vi "SHA1.vi"(1 "String":string) -> (0 "SHA1":string)   [LabVIEW 2023]
panel:
  # "\"\" => da39a3ee5e6b4b0d3255bfef95601890afd80709"
  # "The quick brown fox jumps over the lazy dog =>\n2fd4e1c67a2d28fced849ee1bb76e7391b93eb12"
  # "The quick brown fox jumps over the lazy cog =>\nde9f2c7fd25e1b3afad3e85a0bd17d9b100db4b3"
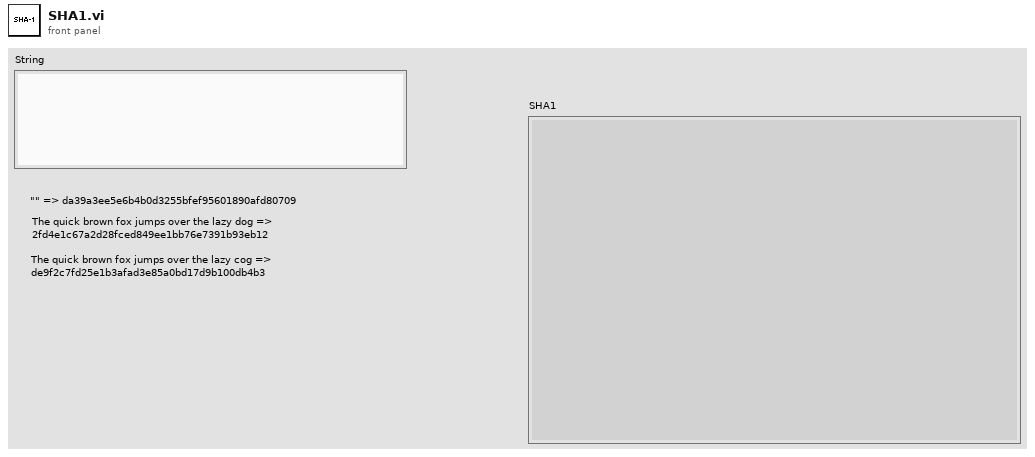
[diagram p1: front panel]
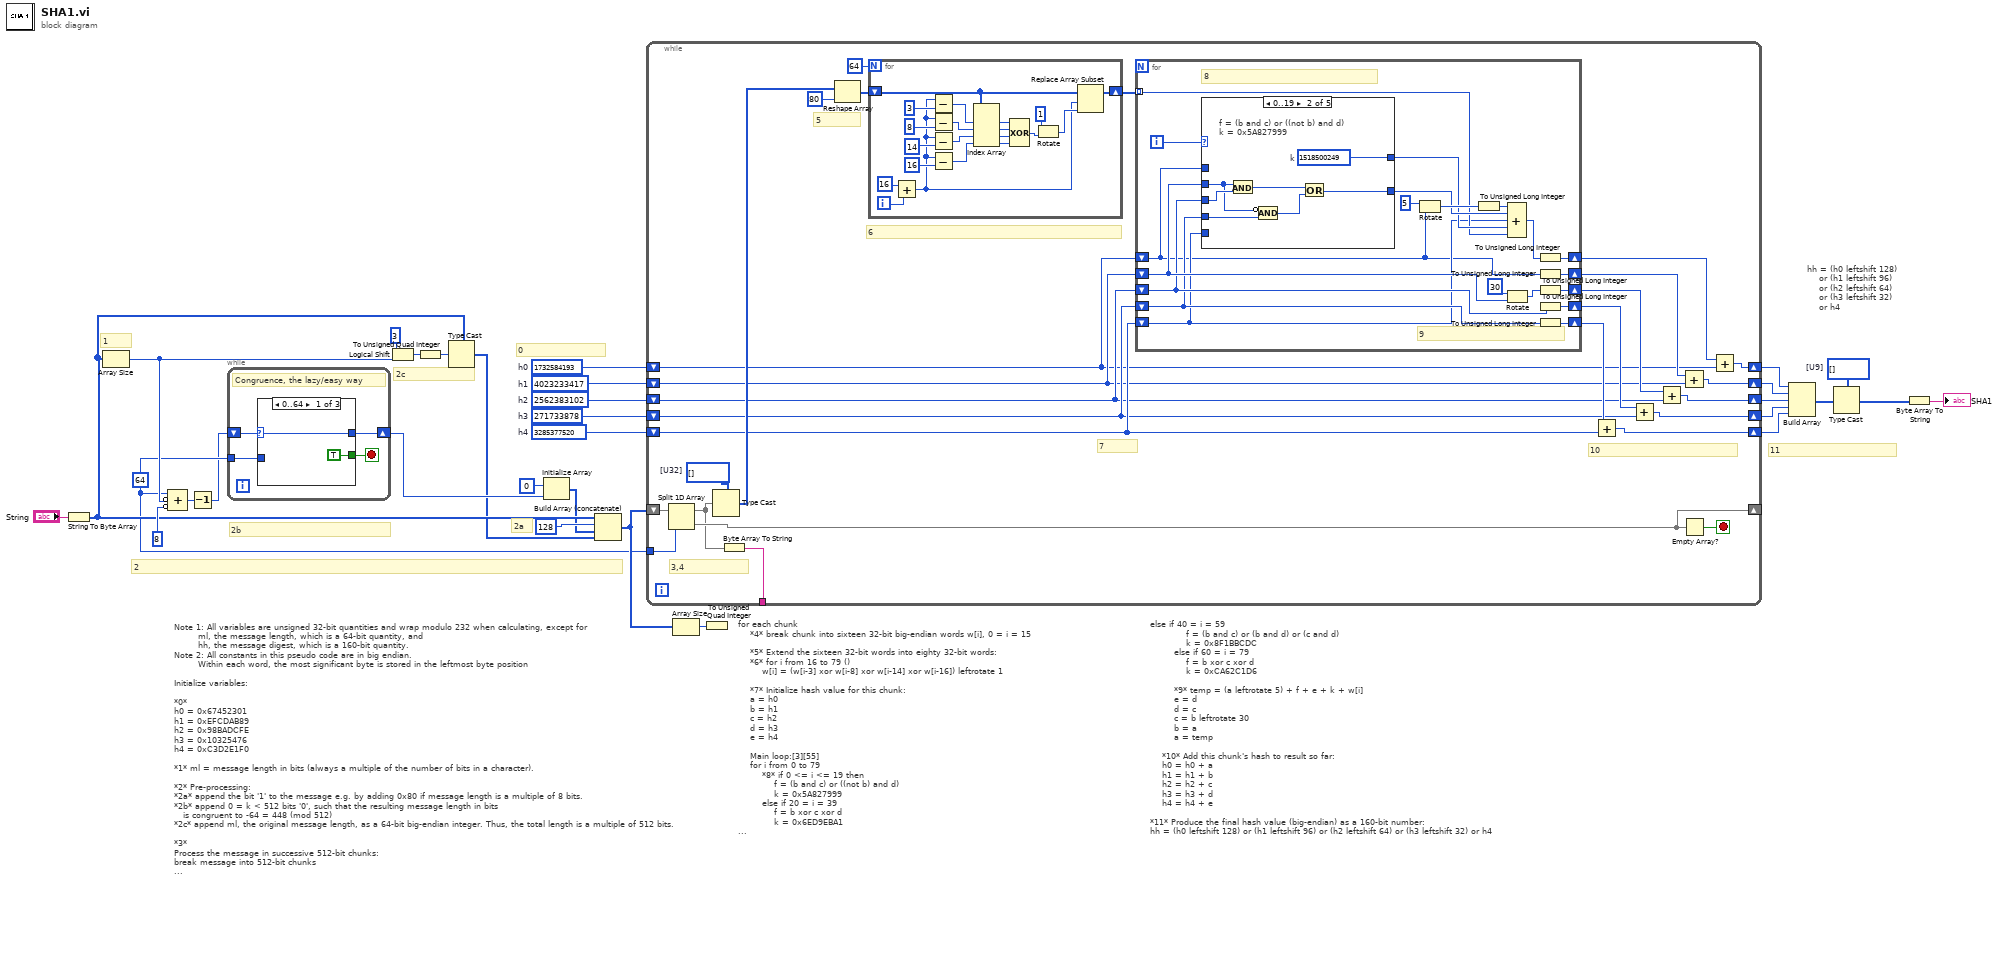
[diagram p0: block diagram]
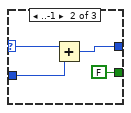
[diagram p2: hidden frame]
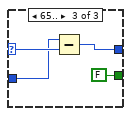
[diagram p3: hidden frame]
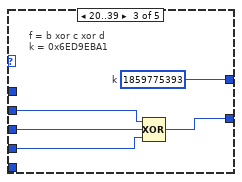
[diagram p5: hidden frame]
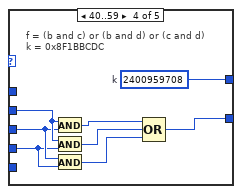
[diagram p6: hidden frame]
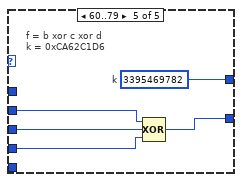
[diagram p7: hidden frame]
diagram:
  w14 = u8[] []  # [U9]
  w4 = 64 ("y")
  w22 = u32 3285377520  # h4
  w23 = u32 271733878  # h3
  w24 = u32 2562383102  # h2
  w25 = u32 4023233417  # h1
  w26 = u32 1732584193  # h0
  # "2c"
  # "2b"
  # "2a"
  # "11"
  # "hh = (h0 leftshift 128) \n    or (h1 leftshift 96) \n    or (h2 leftshift 64) \n    or (h3 leftshift 32) \n    or h4"
  # "2"
  # "1"
  # "0"
  # "else if 40 = i = 59\n            f = (b and c) or (b and d) or (c and d) \n            k = 0x8F1BBCDC\n        else if 60 = i = 79\n            f = b xor c xor d\n            k = 0xCA62C1D6\n\n        *9* temp = (a leftrotate 5) + f + e + k + w[i]\n        e = d\n        d = c\n        c = b leftrotate 30\n        b = a\n        a = temp\n\n    *10* Add this chunk's hash to result so far:\n    h0 = h0 + a\n    h1 = h1 + b \n    h2 = h2 + c\n    h3 = h3 + d\n    h4 = h4 + e\n\n*11* Produce the final hash value (big-endian) as a 160-bit number:\nhh = (h0 leftshift 128) or (h1 leftshift 96) or (h2 leftshift 64) or (h3 leftshift 32) or h4"
  # "for each chunk\n    *4* break chunk into sixteen 32-bit big-endian words w[i], 0 = i = 15\n\n    *5* Extend the sixteen 32-bit words into eighty 32-bit words:\n    *6* for i from 16 to 79 ()\n        w[i] = (w[i-3] xor w[i-8] xor w[i-14] xor w[i-16]) leftrotate 1\n\n    *7* Initialize hash value for this chunk:\n    a = h0\n    b = h1\n    c = h2\n    d = h3\n    e = h4\n\n    Main loop:[3][55]\n    for i from 0 to 79\n        *8* if 0 <= i <= 19 then\n            f = (b and c) or ((not b) and d)\n            k = 0x5A827999\n        else if 20 = i = 39\n            f = b xor c xor d\n            k = 0x6ED9EBA1\n..."
  # "Note 1: All variables are unsigned 32-bit quantities and wrap modulo 232 when calculating, except for\n        ml, the message length, which is a 64-bit quantity, and\n        hh, the message digest, which is a 160-bit quantity.\nNote 2: All constants in this pseudo code are in big endian.\n        Within each word, the most significant byte is stored in the leftmost byte position\n\nInitialize variables:\n\n*0*\nh0 = 0x67452301\nh1 = 0xEFCDAB89\nh2 = 0x98BADCFE\nh3 = 0x10325476\nh4 = 0xC3D2E1F0\n\n*1* ml = message length in bits (always a multiple of the number of bits in a character).\n\n*2* Pre-processing:\n*2a* append the bit '1' to the message e.g. by adding 0x80 if message length is a multiple of 8 bits.\n*2b* append 0 = k < 512 bits '0', such that the resulting message length in bits\n   is congruent to -64 = 448 (mod 512)\n*2c* append ml, the original message length, as a 64-bit big-endian integer. Thus, the total length is a multiple of 512 bits.\n\n*3*\nProcess the message in successive 512-bit chunks:\nbreak message into 512-bit chunks\n..."
  n1 = String To Byte Array(string="String") -> (unsigned byte array=w12:u8[])
  n2 = Array Size(array=w12) -> (size(s)=w5:i32)
  n3 = Compound Arithmetic op=ADD(w4, invert w5, invert 8 ("y")) -> (w30:i32)
  n4 = Decrement(x=w30) -> (x-1=w3:i32)
  n5 = while {
    shift-right: [w33] -> w2
    shift-left: w3 -> [w35]
    tunnel: w4 -> [w34]
    stop <- w32 stop-if-true
    # "Congruence, the lazy/easy way"
    n6 = case shown="0..64" w35 {
      selector: w35 -> [w37 w41 w45]
      tunnel: w34 -> [_ w40 w44]
      tunnel: [w37 w39 w43] -> w33
      tunnel: [TRUE FALSE FALSE] -> w32
      frame 0..64 {
      }
      frame ..-1 {
        n7 = Add(x=w41, y=w40) -> (x+y=w39:i32)
      }
      frame 65.. {
        n8 = Subtract(x=w44, y=w45) -> (x-y=w43:i32)
      }
    }
  }
  n9 = Logical Shift(y=i16 3, x=w5) -> (x << y=w7:i32)
  n10 = To Unsigned Quad Integer(1:w7) -> (0:w28:u64)
  n11 = Type Cast(type=w12, x=w28) -> (*(type *) &x=w1:u8[])
  n12 = Initialize Array(u8 0 ("h0"), w2) -> (w10:u8[])
  n13 = Build Array (concatenate)(w12, u8 128 ("h0"), w10, w1) -> (w9:u8[])
  n14 = while {
    shift-right: [w69] -> _
    shift-left: w9 -> [w72]
    tunnel: w4 -> [w46]
    shift-right: [w68] -> w19
    shift-left: w26 -> [w49]
    shift-right: [w67] -> w18
    shift-left: w25 -> [w50]
    shift-right: [w66] -> w20
    shift-left: w24 -> [w51]
    shift-right: [w65] -> w17
    shift-left: w23 -> [w52]
    shift-right: [w64] -> w21
    shift-left: w22 -> [w53]
    tunnel: [w47] -> _
    stop <- w71 stop-if-true
    w70 = u32[] []  # [U32]
    # "10"
    # "7"
    # "5"
    # "6"
    # "3,4"
    n15 = Split 1D Array(array=w72, index=w46) -> (first subarray=w48:u8[], second subarray=w69:u8[])
    n16 = Type Cast(type=w70, x=w48) -> (*(type *) &x=w58:u32[])
    n17 = Byte Array To String(unsigned byte array=w48) -> (string=w47:string)
    n18 = Reshape Array(w58, 80 ("h0")) -> (w61:u32[])
    n19 = for {
      N: 64 ("h0") -> [_]
      shift-right: [w136] -> w60
      shift-left: w61 -> [w135]
      i -> [w137]
      n20 = Add(x=16 ("h0"), y=w137) -> (x+y=w118:i32)
      n21 = Subtract(x=w118, y=3 ("h0")) -> (x-y=w122:i32)
      n22 = Subtract(x=w118, y=8 ("h0")) -> (x-y=w121:i32)
      n23 = Subtract(x=w118, y=14 ("h0")) -> (x-y=w120:i32)
      n24 = Subtract(x=w118, y=16 ("h0")) -> (x-y=w119:i32)
      n25 = Index Array(array=w135, index #1=w122, index #2=w121, index #3=w120, index #4=w119) -> (element #1=w128:u32, element #2=w129:u32, element #3=w127:u32, element #4=w126:u32)
      n26 = Compound Arithmetic op=XOR(w128, w129, w127, w126) -> (w125:u32)
      n27 = Rotate(1:w125, 2:1 ("h0")) -> (0:w123:u32)
      n28 = Replace Array Subset(array=w135, new element=w123, index=w118) -> (w136:u32[])
    }
    n29 = for {
      tunnel: w60 -> [w88] mode=indexing
      shift-right: [w86] -> w54
      shift-left: w49 -> [w73]
      shift-right: [w82] -> w57
      shift-left: w53 -> [w76]
      shift-right: [w83] -> w59
      shift-left: w52 -> [w77]
      shift-right: [w84] -> w56
      shift-left: w51 -> [w78]
      shift-right: [w85] -> w55
      shift-left: w50 -> [w79]
      i -> [w92]
      # "9"
      # "8"
      n30 = case shown="0..19" w92 {
        tunnel: w73 -> [_ _ _ _ _]
        tunnel: w79 -> [_ w93 w103 w110 w115]
        tunnel: w78 -> [_ w97 w102 w109 w114]
        tunnel: w77 -> [_ w96 w101 w108 w113]
        tunnel: w76 -> [_ _ _ _ _]
        tunnel: [_ w95 w100 w111 w116] -> w90
        tunnel: [_ w94 w104 w112 w117] -> w89
        frame Default {
        }
        frame 0..19 {
          w94 = u32 1518500249  # k
          # "f = (b and c) or ((not b) and d)\nk = 0x5A827999"
          n31 = And(x=w93, y=w97) -> (x .and. y?=w98:u32)
          n32 = Compound Arithmetic op=AND(invert w93, w96) -> (w99:u32)
          n33 = Or(x=w98, y=w99) -> (x .or. y?=w95:u32)
        }
        frame 20..39 {
          w104 = u32 1859775393  # k
          # "f = b xor c xor d\nk = 0x6ED9EBA1"
          n34 = Compound Arithmetic op=XOR(w103, w102, w101) -> (w100:u32)
        }
        frame 40..59 {
          w112 = u32 2400959708  # k
          # "f = (b and c) or (b and d) or (c and d) \nk = 0x8F1BBCDC"
          n35 = And(x=w110, y=w109) -> (x .and. y?=w107:u32)
          n36 = And(x=w110, y=w108) -> (x .and. y?=w106:u32)
          n37 = And(x=w109, y=w108) -> (x .and. y?=w105:u32)
          n38 = Compound Arithmetic op=OR(w107, w106, w105) -> (w111:u32)
        }
        frame 60..79 {
          w117 = u32 3395469782  # k
          # "f = b xor c xor d\nk = 0xCA62C1D6"
          n39 = Compound Arithmetic op=XOR(w115, w114, w113) -> (w116:u32)
        }
      }
      n40 = Rotate(1:w73, 2:5 ("h0")) -> (0:w91:u32)
      n41 = To Unsigned Long Integer(number=w91) -> (unsigned 32bit integer=w75:u32)
      n42 = Rotate(1:w79, 2:30 ("h0")) -> (0:w80:u32)
      n43 = Compound Arithmetic op=ADD(w75, w90, w76, w89, w88) -> (w87:u32)
      n44 = To Unsigned Long Integer(number=w87) -> (unsigned 32bit integer=w86:u32)
      n45 = To Unsigned Long Integer(number=w73) -> (unsigned 32bit integer=w85:u32)
      n46 = To Unsigned Long Integer(number=w80) -> (unsigned 32bit integer=w84:u32)
      n47 = To Unsigned Long Integer(number=w78) -> (unsigned 32bit integer=w83:u32)
      n48 = To Unsigned Long Integer(number=w77) -> (unsigned 32bit integer=w82:u32)
    }
    n49 = Add(x=w57, y=w53) -> (x+y=w64:u32)
    n50 = Add(x=w59, y=w52) -> (x+y=w65:u32)
    n51 = Add(x=w56, y=w51) -> (x+y=w66:u32)
    n52 = Add(x=w55, y=w50) -> (x+y=w67:u32)
    n53 = Empty Array?(array=w69) -> (empty?=w71:bool)
    n54 = Add(x=w54, y=w49) -> (x+y=w68:u32)
  }
  n55 = Array Size(array=w9) -> (size(s)=w8:i32)
  n56 = To Unsigned Quad Integer(1:w8) -> ()  [unwired: 1 out]
  n57 = Build Array(w19, w18, w20, w17, w21) -> (w16:u32[])
  n58 = Type Cast(type=w14, x=w16) -> (*(type *) &x=w13:u8[])
  n59 = Byte Array To String(unsigned byte array=w13) -> (string=→"SHA1":string)
